vi "WFS Get Mla Data 2.vi"(0 "instrument handle":refnum<visa-resource-name>, 7 "MLA Index":i32 format="%.0g", 11 "error in (no error)":errorcluster {"code" format="%.0x"}) -> (1 "Grd Corr Rot":dbl, 2 "Grd Corr 0":dbl, 3 "Spot Offset Y":dbl, 4 "instrument handle out":refnum<visa-resource-name>, 6 "MLA Name":string, 8 "Cam Pitch µm":dbl, 9 "Grd Corr Pitch":dbl, 10 "Lenslet Pitch µm":dbl, 12 "Grd Corr 45":dbl, 13 "Lenslet f µm":dbl, 14 "Spot Offset X":dbl, 15 "error out":errorcluster {"code" format="%.0x"})   [LabVIEW 2020]
doc: "This VI returns calibration data of the desired Microlens Array index. The number of calibrated lenslet arrays can be derived by VI GetMlaCals.\n\nNote: The calibration data are not automatically set active."
uses:
  WFS_32.dll
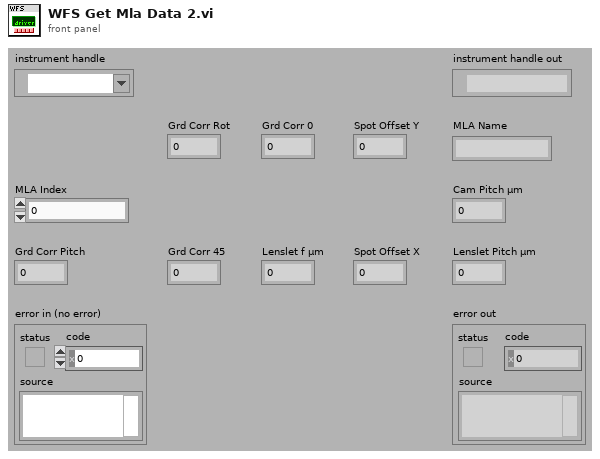
[diagram p1: front panel]
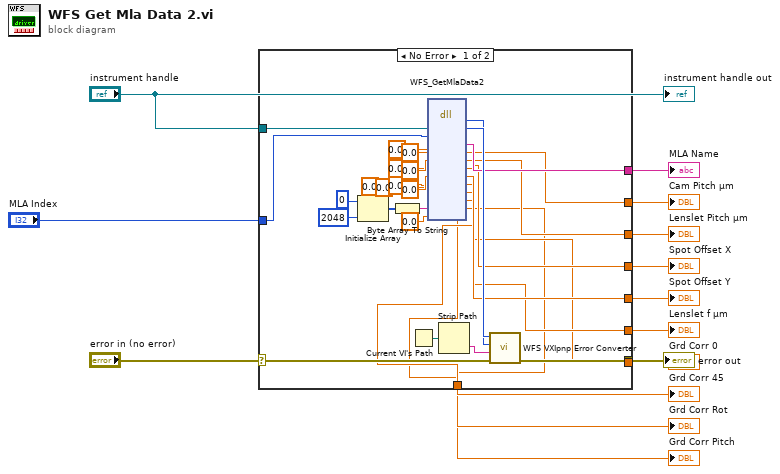
[diagram p0: block diagram]
diagram:
  n1 = case shown="No Error" "error in (no error)" {
    selector: "error in (no error)" -> [w40 w46]
    tunnel: [w39 w46] -> w14
    tunnel: "instrument handle" -> [w44 _]
    tunnel: "MLA Index" -> [w38 _]
    tunnel: [w33 _] -> w10
    tunnel: [w31 _] -> w9
    tunnel: [w29 _] -> w8
    tunnel: [w27 _] -> w7
    tunnel: [w25 _] -> w6
    tunnel: [w23 _] -> w5
    tunnel: [w21 _] -> w4
    tunnel: [w19 _] -> w3
    tunnel: [w17 _] -> w2
    tunnel: [w15 _] -> w1
    frame No Error {
      n2 = Initialize Array(u8 0 ("element"), 2048 ("dimension size")) -> (w36:u8[])
      n3 = Byte Array To String(unsigned byte array=w36) -> (string=w37:string)
      n4 = Current VI's Path() -> (path=w45:path)
      n5 = dll-call lib="WFS_*.*" fn="WFS_GetMlaData2"("Instrument Handle"=w44, "MLA Index"=w38, "MLA Name"=w37, "Cam Pitch µm"=0.0, "Lenslet Pitch µm"=0.0, "Spot Offset X"=0.0, "Spot Offset Y"=0.0, "Lenslet f µm"=0.0, "Grd Corr 0"=0.0, "Grd Corr 45"=0.0, "Grd Corr Rot"=0.0, "Grd Corr Pitch"=0.0) -> (w42:i32, "Instrument Handle"=w43:u32, "MLA Name"=w33:string, "Cam Pitch µm"=w31:dbl, "Lenslet Pitch µm"=w29:dbl, "Spot Offset X"=w27:dbl, "Spot Offset Y"=w25:dbl, "Lenslet f µm"=w23:dbl, "Grd Corr 0"=w21:dbl, "Grd Corr 45"=w19:dbl, "Grd Corr Rot"=w17:dbl, "Grd Corr Pitch"=w15:dbl)  [unwired: 4 in, 2 out]
      n6 = Strip Path(path=w45) -> (name=w41:string)  [unwired: 1 out]
      n7 = call "WFS VXIpnp Error Converter.vi"("error in (no error)"=w40, "Name Of VI (\"\")"=w41, "CVI Error Code (0)"=w42, "instrument handle"=w43) -> ("error out"=w39:errorcluster)  [unwired: 6 in, 1 out]
    }
    frame Error {
    }
  }
  "error out" <- w14
  "MLA Name" <- w10
  "Cam Pitch µm" <- w9
  "Lenslet Pitch µm" <- w8
  "Spot Offset X" <- w7
  "Spot Offset Y" <- w6
  "Lenslet f µm" <- w5
  "Grd Corr 0" <- w4
  "Grd Corr 45" <- w3
  "Grd Corr Rot" <- w2
  "Grd Corr Pitch" <- w1
  "instrument handle out" <- "instrument handle"
